vi "Check Value Type.vi"(8 "error in (no error)":errorcluster, 11 "Column in":refnum<class "Ctrl Refnum Column.lvclass">) -> (0 "error out":errorcluster, 3 "Column out":refnum<class "Ctrl Refnum Column.lvclass">)   [LabVIEW 2020, in "Basic Fields.lvlib" / "Ctrl Refnum Column.lvclass"]
uses:
  Ctrl Refnum Column.lvclass
  Ctrl Refnum Column.lvclass/Ctrl Refnum Column.ctl
  Basic Columns/Basic Columns/Column Class/Column Parent.lvclass
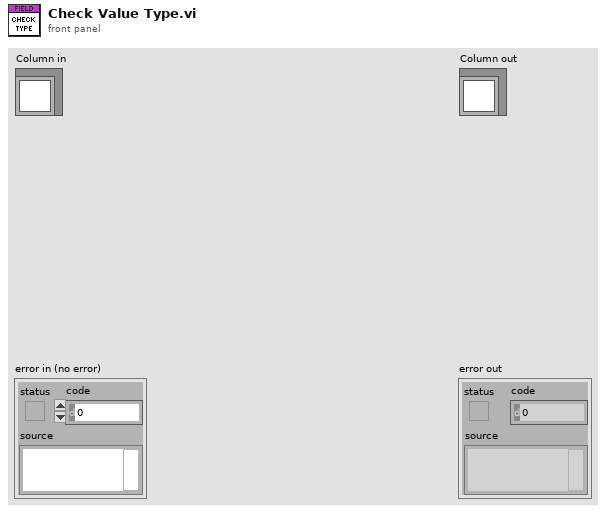
[diagram p1: front panel]
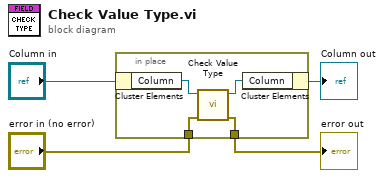
[diagram p0: block diagram]
diagram:
  n1 = in-place {
    in-place-border: "error in (no error)" -> [w6]
    in-place-border: [w5] -> w2
    n2 = in-place-cluster #1("Column in") -> ("Column"=w8:refnum<class "Column Parent.lvclass">)
    n3 = call-dynamic "Check Value Type.vi"("error in (no error)"=w6, "Column in"=w8) -> ("error out"=w5:errorcluster, "Column out"=w7:refnum<class "Column Parent.lvclass">)  [unwired: 8 in]
    n4 = in-place-cluster #1("Column"=w7) -> (→"Column out":refnum<class "Ctrl Refnum Column.lvclass">)
  }
  "error out" <- w2
